vi "CreateDetector.vi"(6 "Detector Settings":T1={"Refine Edges (Default: True)"=TRUE, "Threads (Default: 1)"=1, "Decimate (Default: 1)"=1.0, "Blur (Default: 0)"=0.0, "Bits (Default: 2)"=2} {"Threads (Default: 1)" min=1}, 8 "error in (no error)":errorcluster, 11 "Family":T2) -> (0 "error out":errorcluster, 3 "New ApriltagDetector":refnum<class "AprilTagDetector.lvclass">)   [LabVIEW 2020, in "g_ar_toolkit.feature_detection.lvlib" / "AprilTagDetector.lvclass"]
uses:
  AprilTagDetector.lvclass
  AprilTag Families.ctl
  Detector Settings.ctl
  AprilTagDetector.lvclass/AprilTagDetector.ctl
  g_ar_toolkit.common/g_ar_toolkit.common.lvlib
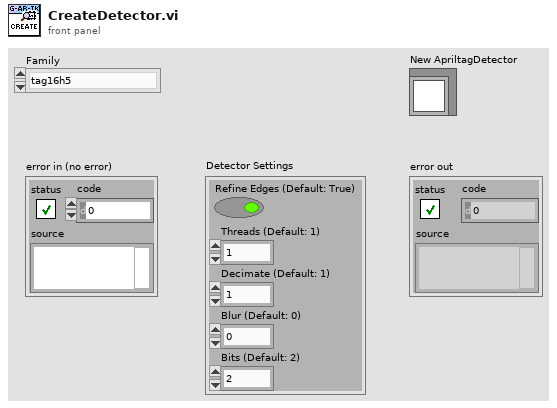
[diagram p1: front panel]
types:
  T1 = typedef "g_ar_toolkit.feature_detection.lvlib/AprilTagDetector.lvclass/Detector Settings.ctl" = cluster{"Refine Edges (Default: True)":bool, "Threads (Default: 1)":u8, "Decimate (Default: 1)":sgl, "Blur (Default: 0)":sgl, "Bits (Default: 2)":u8}
  T2 = typedef "g_ar_toolkit.feature_detection.lvlib/AprilTagDetector.lvclass/AprilTag Families.ctl" = enum8{"tag16h5", "tag25h9", "tag36h11", "tagCircle21h7", "tagCircle49h12", "tagCustom48h12", "tagStandard41h12", "tagStandard52h13"}
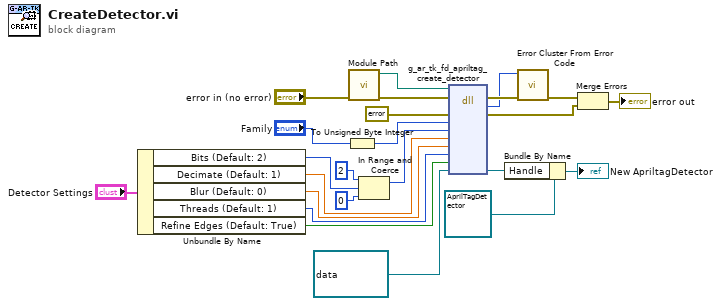
[diagram p0: block diagram]
diagram:
  n1 = Unbundle By Name("Detector Settings") -> ("Bits (Default: 2)"=w5:u8, "Decimate (Default: 1)"=w6:sgl, "Blur (Default: 0)"=w7:sgl, "Threads (Default: 1)"=w8:u8, "Refine Edges (Default: True)"=w9:bool)
  n2 = To Unsigned Byte Integer(number="Family") -> (unsigned 8bit integer=w14:u8)
  n3 = call "Module Path.vi"("error in (no error)"="error in (no error)") -> ("error out"=w2:errorcluster, "Path"=w1:path)  [unwired: 9 in]
  n4 = In Range and Coerce(upper limit=u8 2, x=w5, lower limit=u8 0) -> (coerced(x)=w13:u8)  [unwired: 1 out]
  n5 = dll-call lib="?" fn="g_ar_tk_fd_apriltag_create_detector" ("g_ar_toolkit.*.*:g_ar_tk_capture_context_create")(path in=w1, error in=w2, "error_cluster"=errorcluster {"status"=FALSE, "code"=0, "source"=""} ("error constant"), "tag_family"=w14, "bits"=w13, "decimate"=w6, "blur"=w7, "threads"=w8, "refine_edges"=w9, "EDVR"=refnum<data-value> refnum) -> (error out=w23:errorcluster, "MgErr"=w22:i32, "error_cluster"=w19:errorcluster, "EDVR"=w17:refnum<data-value>)  [unwired: 7 in, 1 out]
  n6 = Bundle By Name(cluster=refnum<class "AprilTagDetector.lvclass"> refnum ("CameraManager out"), "Handle"=w17) -> (→"New ApriltagDetector":refnum<class "AprilTagDetector.lvclass">)
  n7 = call <vilib>:"Error Cluster From Error Code.vi"("error in (no error)"=w23, "error code (0)"=w22) -> ("error out"=w21:errorcluster)  [unwired: 7 in]
  n8 = Merge Errors(w21, w19) -> (→"error out":errorcluster)
